vi "RT_Main_JC.vi"() -> ()   [LabVIEW 2018]
uses:
  Type Defs/voltage range.ctl
  Type Defs/write file states.ctl
  Type Defs/ramp parameters.ctl
  Type Defs/ramp states.ctl
  <vilib>/Platform/TimedLoop/XDataNode/timing_clust.ctl
  <vilib>/Platform/TimedLoop/XDataNode/nitl_modes.ctl
  <vilib>/Platform/TimedLoop/XDataNode/wakeup.ctl
  Type Defs/Calibration Values.ctl
  RT All Loop Stop.vi
  <vilib>/FPGAPlugInAG/myRIO-1900/niLvFpga_Open_myRIO-1900.vi
  <vilib>/rvi/interface/common/dynamic/niFpgaDynamicAddResources.vi
  <vilib>/Utility/error.llb/Error Cluster From Error Code.vi
  <vilib>/rvi/errors/niLvFpgaAdjustHostInterfaceError.vi
  <vilib>/rvi/interface/common/niFpgaWaitOnOcc.vi
  <vilib>/FPGAPlugInAG/Dynamic/niLvFpga_Close_Dynamic.vi
  <vilib>/Platform/TimedLoop/XDataNode/XDataNode.xnode
  <vilib>/rvi/interface/nirviOpenFPGA/nirviOpenFPGA.xnode
  FPGA Bitfiles/focus-probe-meas_FPGATarget_FPGAMain_5fPMfgVhfVY.lvbitx
  FPGA_Main_TeamUNCC.vi
  <vilib>/rvi/interface/nirviReadWriteControl/nirviReadWriteControl.xnode
  <vilib>/rvi/interface/nirviMethod/nirviMethod.xnode
  <vilib>/rvi/interface/nirviCloseFPGA/nirviCloseFPGA.xnode
  <vilib>/rvi/interface/Simulation/niFpgaSimulationCallBeginRW.vi
  <vilib>/Platform/TimedLoop/XDataNode/XDNodeRunTimeDep.lvlib
  NiFpgaLv.dll
  <vilib>/FPGAPlugInAG/Dynamic/niLvFpga_ConfigureFifo_Dynamic.vi
  <vilib>/rvi/errors/niLvFpgaMergeErrorWithErrorCode.vi
panel:
  out "Measurement States":enum16{"Idle", "Align", "Measure"}(ring)
  in  "ramp down multiplier":i32=1
  in  "Voltage Range":T1={"Vmax"=2700, "Vmin"=1800}
  in  "Total Ramp Time (us)":i64=5000000
  out "Elements in Queue":i32
  out "Writing?":bool
  out "Measuring?":bool
  out "Late?":bool=TRUE
  out "Overflow?":bool=TRUE
  out "VC Voltage Out":u16=1350
  out "dV":u16=65535
  out "to RT - elements \nremaining":u32
  in  "number of elements\nto read from FPGA":u32=1500
  out "from FPGA:\nactual depth":u32=4096
  in  "FPGA Rate (kS/s)":sgl=50.0
  out "FPGA Period (ms)":sgl=0.02
  in  "stop":bool
  in  "RT loop time (us)":i64=5000
  out "RT loop rate (kHz)":dbl=6.961933457817009
  out "RT Loop Rate (ms)":u32
  # "Ramp"
  # "Status"
  # "FPGA Parameters"
  # "FPGA Loop Speed"
  # "RT Loop Speed"
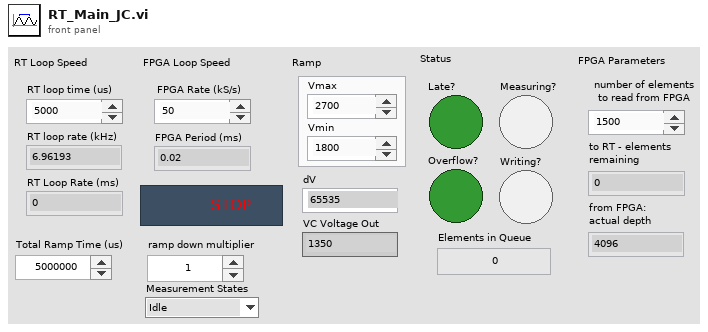
[diagram p1: front panel]
types:
  T1 = typedef "voltage range.ctl" = cluster{"Vmax":u16, "Vmin":u16}
  T2 = typedef "ramp parameters.ctl" = cluster{"Ramp State":T3, "Ramp dV":u16, "Ramp Voltage":u16}
  T3 = typedef "ramp states.ctl" = enum16{"intialize", "Ramp Down", "ramp up", "max"}
  T4 = typedef "write file states.ctl" = enum16{"idle", "create file", "write data", "close file"}
  T5 = enum16{"open", "replace", "create", "open or create", "replace or create", "replace or create with confirmation"}
  T6 = typedef "XDNodeRunTimeDep.lvlib/timing_clust.ctl" = cluster{"Expected End [f-1]":u64, "Actual End [f-1]":u64, "Finished Late? [f-1]":bool, "Expected End [i-1]":u64, "Actual End [i-1]":u64, "Finished Late? [i-1]":bool, "Expected Start [i]":u64, "Actual Start [i]":u64, "Expected Start [f]":u64, "Actual Start [f]":u64, "Source Name":string, "Structure Name":string, "Period":i64, "Deadline":i64, "Offset":i64, "Start":i64, "Priority":i32, "Timeout":i32, "Mode":T7, "Wakeup Reason":T8, "Error":errorcluster, "Source Type":string, "Secondary Source Type":string, "Global End Time":u64, "Global Start Time":u64, "Frame Duration":u64, "Iteration Duration":u64, "Assigned CPU":i32, "I/O Scan Engine Mode":u32}
  T7 = typedef "XDNodeRunTimeDep.lvlib/nitl_modes.ctl" = enum32{"No Change", "Process missed periods, maintain original phase", "Discard missed periods, maintain original phase", "Process missed periods, ignore original phase", "Discard missed periods, ignore original phase"}
  T8 = typedef "XDNodeRunTimeDep.lvlib/wakeup.ctl" = enum32{"Normal", "Aborted", "Asynchronous wakeup", "Timing source error", "Timed loop error", "Timeout"}
  T9 = typedef "Calibration Values.ctl" = cluster{"cap probe":i16, "photodetector":i16, "knife edge sensor":i16, "Ramp Voltage":u16}
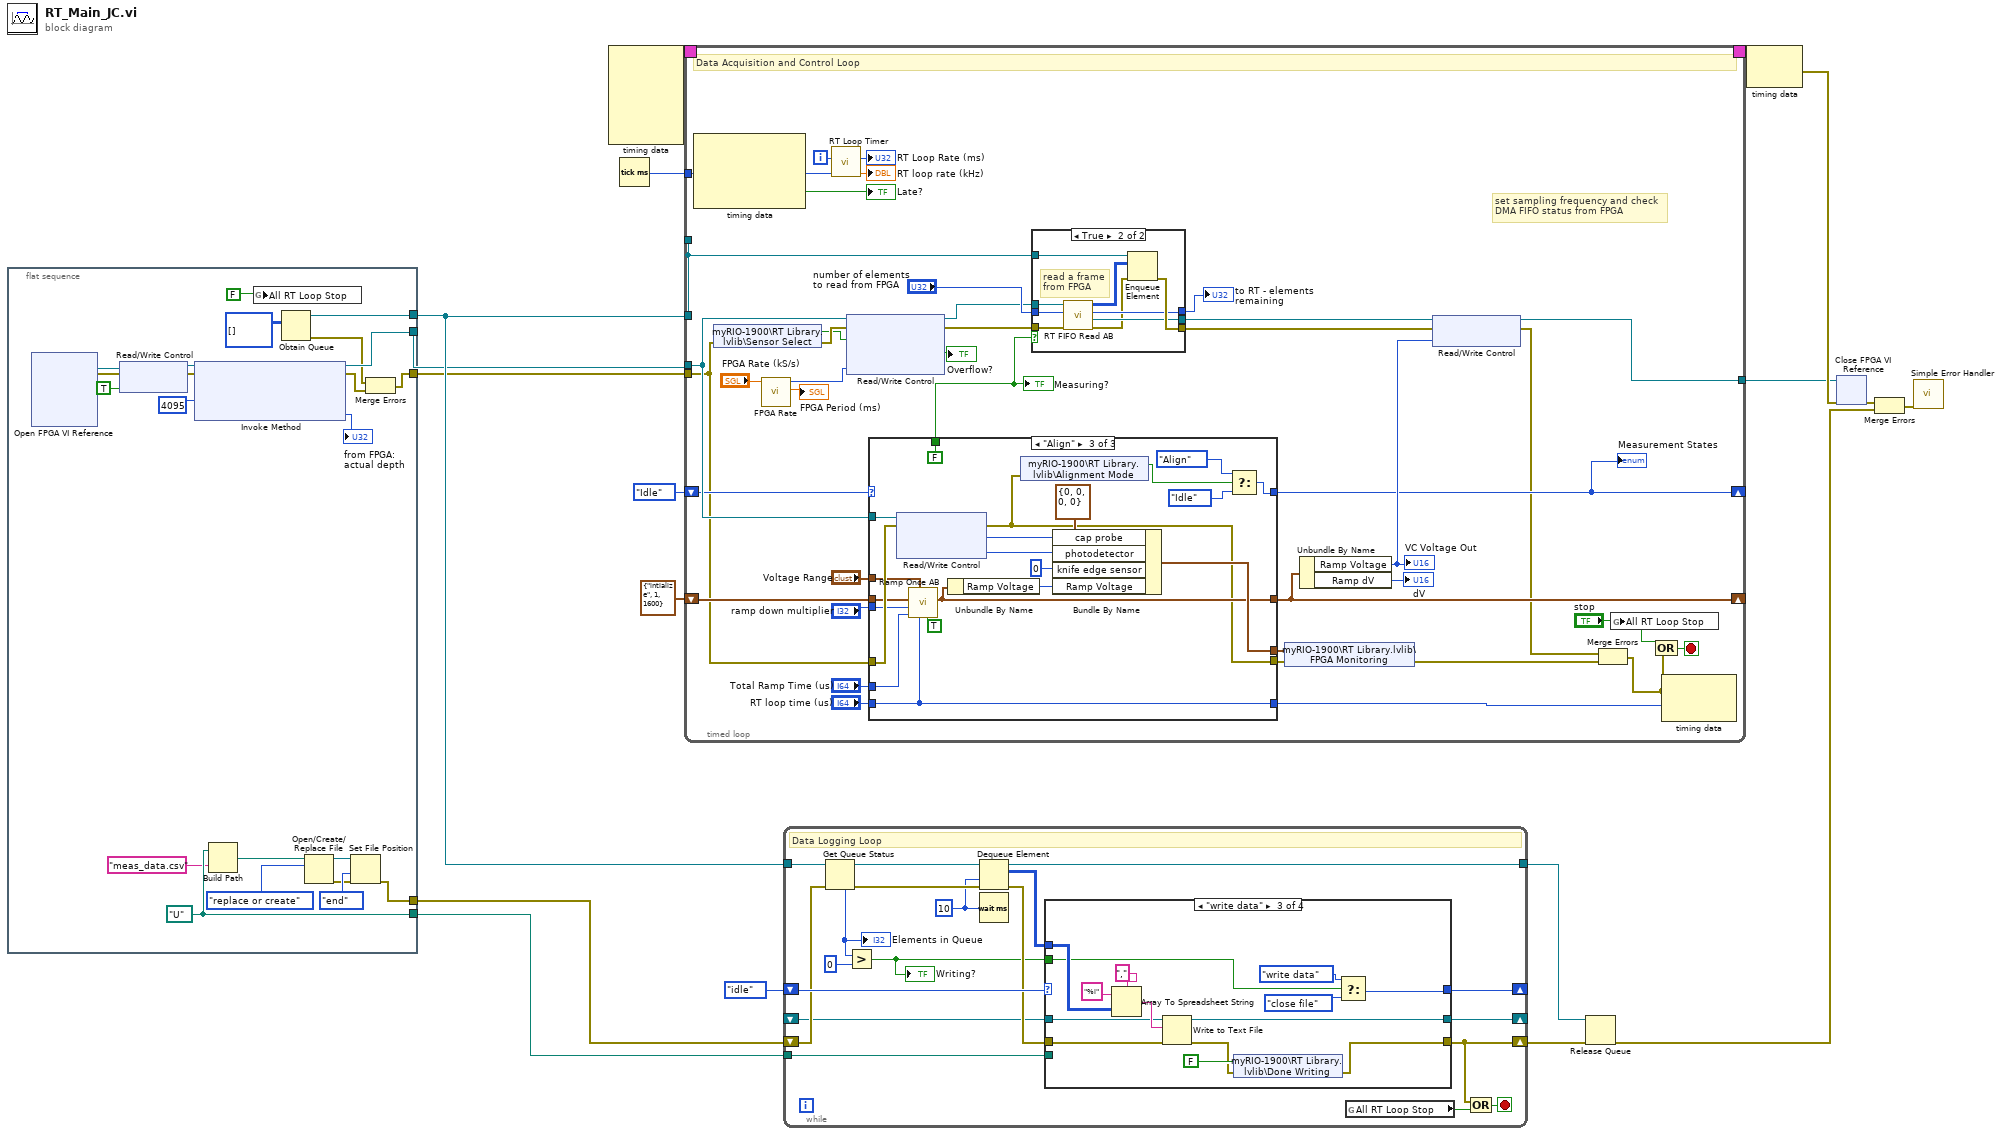
[diagram p0: block diagram]
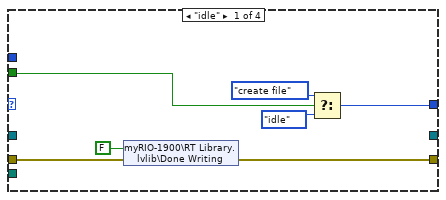
[diagram p2: hidden frame]
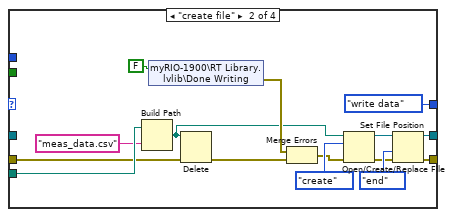
[diagram p3: hidden frame]
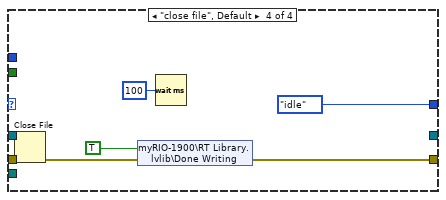
[diagram p4: hidden frame]
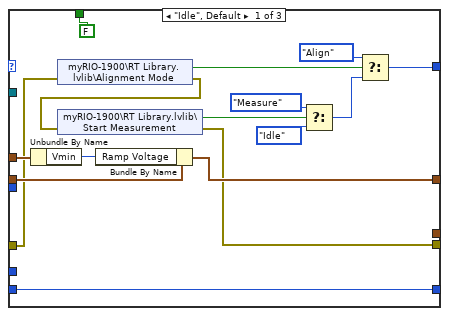
[diagram p5: hidden frame]
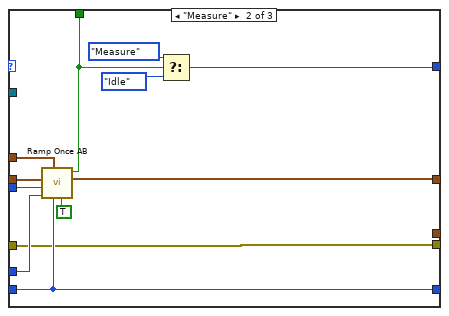
[diagram p6: hidden frame]
diagram:
  n1 = flat-sequence {
    tunnel: [w39] -> w3
    tunnel: [w36] -> w7
    tunnel: [w34] -> w13
    tunnel: [w28] -> w6
    tunnel: [w26] -> w5
    frame #0 {
      w28 = path "U:/" ("USB flash drive")
      n2 = xnode "Open FPGA VI Reference"() -> ("FPGA VI Reference Out"=w20:refnum<k20>, "error out"=w19:errorcluster)  [unwired: 2 in]
      n3 = xnode "Read/Write Control"("FPGA VI Reference In"=w20, "error in"=w19, "amplifier"=TRUE ("amplifier  (F = ENABLE)")) -> ("FPGA VI Reference Out"=w23:refnum<k20>, "error out"=w22:errorcluster)
      n4 = xnode "Invoke Method"("FPGA VI Reference In"=w23, "error in"=w22, "Requested Depth"=u32 4095) -> ("FPGA VI Reference Out"=w39:refnum<k20>, "error out"=w37:errorcluster, "Actual Depth"=→"from FPGA:\nactual depth":u32)
      n5 = Build Path(base path=w28, name or relative path="meas_data.csv") -> (appended path=w25:path)
      n6 = global write "RT All Loop Stop.vi" "All RT Loop Stop"(FALSE ("Abort")) -> ()
      n7 = Obtain Queue(element data type=i16[][] [] ("transposed array")) -> (queue out=w34:refnum<queue>, error out=w21:errorcluster)  [unwired: 4 in, 1 out]
      n8 = Open/Create/Replace File(file path (use dialog)=w25, operation (0:open)=T5."replace or create") -> (refnum out=w31:refnum<file>, error out=w29:errorcluster)  [unwired: 4 in, 1 out]
      n9 = Set File Position(refnum=w31, from (0:start)=enum16{"start", "end", "current"}."end", error in=w29) -> (error out=w26:errorcluster)  [unwired: 1 in, 1 out]
      n10 = Merge Errors(w21, w37) -> (w36:errorcluster)
    }
  }
  n11 = node-c288() -> (w16:T6)  [unwired: 5 in]
  n12 = Tick Count (ms)() -> (millisecond timer value=w14:u32)
  n13 = timed-loop {
    tunnel: w3 -> [w54]
    tunnel: w7 -> [w44]
    timing: w16 -> [_]
    timing-out: [_] -> w15
    tunnel: w14 -> [w71]
    tunnel: w13 -> [w67]
    tunnel: [w67] -> _
    tunnel: [w64] -> w4
    shift-right: [w53] -> _
    shift-left: T2 {"Ramp State"=enum."intialize", "Ramp dV"=1, "Ramp Voltage"=1600} ("Parameters") -> [w56]
    shift-right: [w48] -> _
    shift-left: enum16{"Idle", "Align", "Measure"}."Idle" ("Measurement States 2") -> [w52]
    i -> [w72]
    stop <- w78 stop-if-true
    # "set sampling frequency and check\nDMA FIFO status from FPGA"
    # "Data Acquisition and Control Loop"
    n14 = node-c288() -> (→"Late?":bool)  [unwired: 1 in, 3 out]
    n15 = shared-variable "myRIO-1900\\RT Library.lvlib\\Sensor Select"(error in=w44) -> (w41:bool, error out=w43:errorcluster)
    n16 = call "FPGA Rate.vi"("FPGA Rate (kS/s)"="FPGA Rate (kS/s)") -> ("FPGA Period (ms)"=→"FPGA Period (ms)":sgl, "FPGA Period(us)"=w42:u32)  [unwired: 9 in]
    n17 = call "RT Loop Timer.vi"("start time"=w71, "loop counter"=w72) -> ("RT loop rate (kHz)"=→"RT loop rate (kHz)":dbl, "RT Loop Rate (ms)"=→"RT Loop Rate (ms)":u32)  [unwired: 8 in]
    n18 = xnode "Read/Write Control"("FPGA VI Reference In"=w54, "error in"=w43, "sensor select"=w41, "loop time (us)"=w42) -> ("FPGA VI Reference Out"=w63:refnum<k20>, "error out"=w74:errorcluster, "Overflow to RT?"=→"Overflow?":bool)
    n19 = case shown="\"Align\"" w52 {
      tunnel: [FALSE w99 FALSE] -> w59
      tunnel: w44 -> [w82 w102 w125]
      tunnel: [w87 w102 w110] -> w47
      tunnel: "Total Ramp Time (us)" -> [_ w107 w129]
      tunnel: "RT loop time (us)" -> [w92 w106 w128]
      tunnel: [w93 w108 w116] -> w53
      tunnel: [w92 w106 w128] -> w60
      tunnel: "Voltage Range" -> [w96 w105 w124]
      tunnel: w56 -> [w95 w104 w123]
      tunnel: "ramp down multiplier" -> [_ w103 w122]
      tunnel: w54 -> [_ _ w119]
      tunnel: [_ _ w117] -> w51
      tunnel: [w83 w98 w112] -> w48
      frame "Idle", Default {
        n20 = Unbundle By Name(w96) -> ("Vmin"=w94:u16)
        n21 = shared-variable "myRIO-1900\\RT Library.lvlib\\Alignment Mode"(error in=w82) -> (w84:bool, error out=w81:errorcluster)
        n22 = shared-variable "myRIO-1900\\RT Library.lvlib\\Start Measurement"(error in=w81) -> (w91:bool, error out=w87:errorcluster)
        n23 = Bundle By Name(cluster=w95, "Ramp Voltage"=w94) -> (w93:T2)
        n24 = Select(t=enum16{"Idle", "Align", "Measure"}."Measure" ("Measurement States 2"), s=w91, f=enum16{"Idle", "Align", "Measure"}."Idle" ("Measurement States 2")) -> (s? t:f=w85:enum16{"Idle", "Align", "Measure"})
        n25 = Select(t=enum16{"Idle", "Align", "Measure"}."Align" ("Measurement States 2"), s=w84, f=w85) -> (s? t:f=w83:enum16{"Idle", "Align", "Measure"})
      }
      frame "Measure" {
        n26 = call "Ramp Once AB.vi"("start ramp"=TRUE, "RT Loop Time (us)"=w106, "Voltage range"=w105, "Total Ramp Time (us)"=w107, "down ramp multiplier"=w103, "Parameters In"=w104) -> ("Parameters Out"=w108:T2, "Measuring?"=w99:bool)  [unwired: 4 in]
        n27 = Select(t=enum16{"Idle", "Align", "Measure"}."Measure" ("Measurement States 2"), s=w99, f=enum16{"Idle", "Align", "Measure"}."Idle" ("Measurement States 2")) -> (s? t:f=w98:enum16{"Idle", "Align", "Measure"})
      }
      frame "Align" {
        n28 = xnode "Read/Write Control"("FPGA VI Reference In"=w119, "error in"=w125) -> ("error out"=w110:errorcluster, "cap probe"=w111:i16, "photodetector"=w127:i16)  [unwired: 1 out]
        n29 = call "Ramp Once AB.vi"("start ramp"=TRUE, "RT Loop Time (us)"=w128, "Voltage range"=w124, "Total Ramp Time (us)"=w129, "down ramp multiplier"=w122, "Parameters In"=w123) -> ("Parameters Out"=w116:T2)  [unwired: 4 in, 1 out]
        n30 = Unbundle By Name(w116) -> ("Ramp Voltage"=w118:u16)
        n31 = shared-variable "myRIO-1900\\RT Library.lvlib\\Alignment Mode"(error in=w110) -> (w115:bool)  [unwired: 1 out]
        n32 = Bundle By Name(cluster=T9 {"cap probe"=0, "photodetector"=0, "knife edge sensor"=0, "Ramp Voltage"=0} ("output cluster"), "cap probe"=w111, "photodetector"=w127, "knife edge sensor"=0, "Ramp Voltage"=w118) -> (w117:T9)
        n33 = Select(t=enum16{"Idle", "Align", "Measure"}."Align" ("Measurement States 2"), s=w115, f=enum16{"Idle", "Align", "Measure"}."Idle" ("Measurement States 2")) -> (s? t:f=w112:enum16{"Idle", "Align", "Measure"})
      }
    }
    "Measuring?" <- w59
    "Measurement States" <- w48
    n34 = case shown="True" w59 {
      tunnel: [w137 w146] -> w58
      tunnel: w67 -> [_ w145]
      tunnel: "number of elements\nto read from FPGA" -> [_ w144]
      tunnel: w74 -> [w137 w143]
      tunnel: w63 -> [w136 w138]
      tunnel: [w136 w142] -> w65
      tunnel: [_ w140] -> w73
      frame False {
      }
      frame True {
        # "read a frame from FPGA"
        n35 = call "RT FIFO Read AB.vi"("error in"=w143, "Elements to Read"=w144, "FPGA VI Reference In"=w138) -> ("error out"=w139:errorcluster, "FPGA VI Reference Out"=w142:refnum<k20>, "to RT - elements \nremaining"=w140:u32, "data"=w141:i16[][])  [unwired: 5 in]
        n36 = Enqueue Element(queue=w145, element=w141, error in (no error)=w139) -> (error out=w146:errorcluster)  [unwired: 1 in, 2 out]
      }
    }
    "to RT - elements \nremaining" <- w73
    n37 = shared-variable "myRIO-1900\\RT Library.lvlib\\FPGA Monitoring"(w51, error in=w47) -> (error out=w45:errorcluster)
    n38 = Unbundle By Name(w53) -> ("Ramp Voltage"=w49:u16, "Ramp dV"=→"dV":u16)
    "VC Voltage Out" <- w49
    n39 = xnode "Read/Write Control"("FPGA VI Reference In"=w65, "error in"=w58, "voltage to v.c."=w49) -> ("FPGA VI Reference Out"=w64:refnum<k20>, "error out"=w46:errorcluster)
    n40 = Merge Errors(w46, w45) -> (w66:errorcluster)
    n41 = global write "RT All Loop Stop.vi" "All RT Loop Stop"("stop") -> ()
    n42 = Compound Arithmetic op=OR("stop", w66) -> (w78:bool)
    n43 = node-c288(w66, w60) -> ()  [unwired: 1 out]
  }
  n44 = while {
    tunnel: w13 -> [w163]
    tunnel: [w165] -> w10
    shift-right: [w156] -> _
    shift-left: write_file_states."idle" -> [w157]
    shift-right: [w155] -> _
    shift-left: _ -> [w147]
    shift-right: [w150] -> w8
    shift-left: w5 -> [w153]
    tunnel: w6 -> [w148]
    stop <- w164 stop-if-true
    w158 = 10 ("timeout in ms (-1)")
    # "Data Logging Loop"
    n45 = Get Queue Status(queue=w163, error in (no error)=w153) -> (queue out=w162:refnum<queue>, error out=w161:errorcluster, # elements in queue=w149:i32)  [unwired: 1 in, 5 out]
    "Elements in Queue" <- w149
    n46 = Greater?(x=w149, y=0) -> (0:w151:bool)
    "Writing?" <- w151
    n47 = Dequeue Element(queue=w162, timeout in ms (-1)=w158, error in (no error)=w161) -> (queue out=w165:refnum<queue>, element=w154:i16[][], error out=w152:errorcluster)  [unwired: 1 out]
    n48 = Wait (ms)(milliseconds to wait=w158) -> ()  [unwired: 1 out]
    n49 = case shown="\"write data\"" w157 {
      tunnel: [w172 write_file_states."write data" w198 write_file_states."idle"] -> w156
      tunnel: w151 -> [w169 _ w193 _]
      tunnel: [_ w183 w192 _] -> w155
      tunnel: w152 -> [w167 w178 w194 w207]
      tunnel: [w166 w181 w188 w204] -> w150
      tunnel: w154 -> [_ _ w195 _]
      tunnel: w148 -> [_ w180 _ _]
      tunnel: w147 -> [_ _ w191 w203]
      frame "idle" {
        n50 = shared-variable "myRIO-1900\\RT Library.lvlib\\Done Writing"(FALSE, error in=w167) -> (error out=w166:errorcluster)
        n51 = Select(t=write_file_states."create file", s=w169, f=write_file_states."idle") -> (s? t:f=w172:T4)
      }
      frame "create file" {
        n52 = Build Path(base path=w180, name or relative path="meas_data.csv") -> (appended path=w173:path)
        n53 = shared-variable "myRIO-1900\\RT Library.lvlib\\Done Writing"(FALSE) -> (error out=w176:errorcluster)  [unwired: 1 in]
        n54 = Delete(path (use dialog)=w173, error in=w178) -> (error out=w175:errorcluster)  [unwired: 3 in, 2 out]
        n55 = Merge Errors(w176, w175) -> (w177:errorcluster)
        n56 = Open/Create/Replace File(file path (use dialog)=w173, error in=w177, operation (0:open)=T5."create") -> (refnum out=w186:refnum<file>, error out=w184:errorcluster)  [unwired: 3 in, 1 out]
        n57 = Set File Position(refnum=w186, from (0:start)=enum16{"start", "end", "current"}."end", error in=w184) -> (refnum out=w183:refnum<file>, error out=w181:errorcluster)  [unwired: 1 in]
      }
      frame "write data" {
        n58 = Array To Spreadsheet String(delimiter (Tab)=",", array=w195, 3:"%i" ("format string")) -> (spreadsheet string=w199:string)
        n59 = Write to Text File(file (use dialog)=w191, text=w199, error in=w194) -> (refnum out=w192:refnum<file>, error out=w189:errorcluster)  [unwired: 1 in, 1 out]
        n60 = shared-variable "myRIO-1900\\RT Library.lvlib\\Done Writing"(FALSE, error in=w189) -> (error out=w188:errorcluster)
        n61 = Select(t=write_file_states."write data", s=w193, f=write_file_states."close file") -> (s? t:f=w198:T4)
      }
      frame "close file", Default {
        n62 = Close File(refnum=w203, error in=w207) -> (error out=w205:errorcluster)  [unwired: 1 out]
        n63 = shared-variable "myRIO-1900\\RT Library.lvlib\\Done Writing"(TRUE, error in=w205) -> (error out=w204:errorcluster)
        n64 = Wait (ms)(milliseconds to wait=u32 100) -> ()  [unwired: 1 out]
      }
    }
    n65 = global read "RT All Loop Stop.vi" "All RT Loop Stop"() -> (w159:bool)
    n66 = Compound Arithmetic op=OR(w150, w159) -> (w164:bool)
  }
  n67 = Release Queue(queue=w10, error in (no error)=w8) -> (error out=w11:errorcluster)  [unwired: 1 in, 2 out]
  n68 = node-c288(w15) -> (w12:errorcluster)
  n69 = xnode "Close FPGA VI Reference"("FPGA VI Reference In"=w4, "error in"=w12) -> ("error out"=w18:errorcluster)
  n70 = Merge Errors(w18, w11) -> (w17:errorcluster)
  n71 = call <vilib>:"Simple Error Handler.vi"("error in (no error)"=w17) -> ()  [unwired: 4 in, 5 out]
